vi "Initialize.vi"(8 "error in (no error)":errorcluster, 11 "Thread in":refnum<class "Thread.lvclass">) -> (0 "error out":errorcluster, 3 "Thread out":refnum<class "Thread.lvclass">)   [LabVIEW 2017, in "DSF Core.lvlib" / "Thread.lvclass"]
uses:
  Thread.lvclass
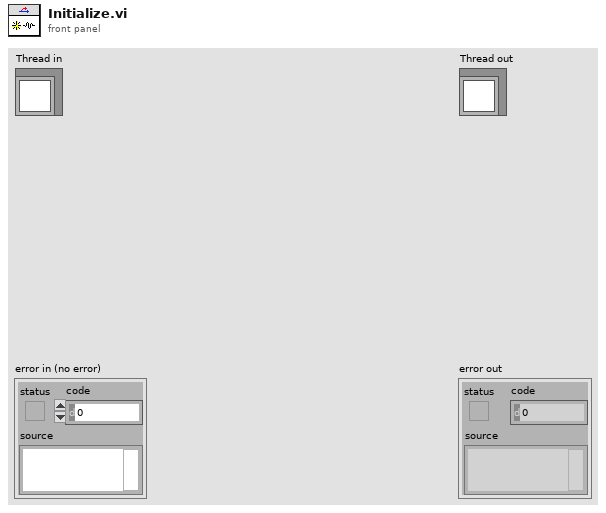
[diagram p1: front panel]
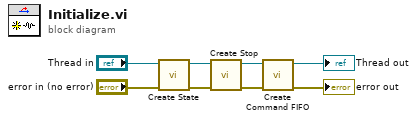
[diagram p0: block diagram]
diagram:
  n1 = call "Create State.vi"("error in (no error)"="error in (no error)", "Thread in"="Thread in") -> ("error out"=w5:errorcluster, "Thread out"=w4:refnum<class "Thread.lvclass">)  [unwired: 8 in]
  n2 = call "Create Stop.vi"("error in (no error)"=w5, "Thread in"=w4) -> ("error out"=w6:errorcluster, "Thread out"=w7:refnum<class "Thread.lvclass">)  [unwired: 8 in]
  n3 = call "Create Command FIFO.vi"("error in (no error)"=w6, "Thread in"=w7) -> ("error out"=→"error out":errorcluster, "Thread out"=→"Thread out":refnum<class "Thread.lvclass">)  [unwired: 8 in]
